vi "Get SubpanelVI Info.vi"(8 "error in (no error)":errorcluster, 11 "Motor Configuration in":refnum<class "LogicIO Configuration.lvclass">) -> (0 "error out":errorcluster, 1 "Subpanel VI data":T1, 2 "Category string":string, 3 "Motor Configuration out":refnum<class "LogicIO Configuration.lvclass">)   [LabVIEW 2016, in "Hardware.lvlib" / "LogicIO.lvlib" / "LogicIO Configuration.lvclass"]
uses:
  <userlib>/Common Components/Hardware/LogicIO/LogicIO Config/LogicIO Configuration.lvclass
  <userlib>/Configuration Dialog Actor/Methods/Data Retrieved by Lookup Table.ctl
  <userlib>/Configuration Dialog Actor/Configuration.lvclass
  <userlib>/Common Components/Hardware/LogicIO/LogicIO Config/LogicIO Configuration.lvclass/LogicIO Configuration.ctl
  <userlib>/Common Components/Hardware/Abstract Hardware/Hardware.lvclass/Hardware.ctl
  <userlib>/Common Components/Hardware/Abstract Hardware/Read Label.vi
  <userlib>/Common Components/Hardware/LogicIO/LogicIO/LogicIO.lvclass
  C:/Program Files (x86)/National Instruments/LabVIEW 2016/user.lib/Common Components/Hardware/Abstract Hardware/Hardware.lvclass
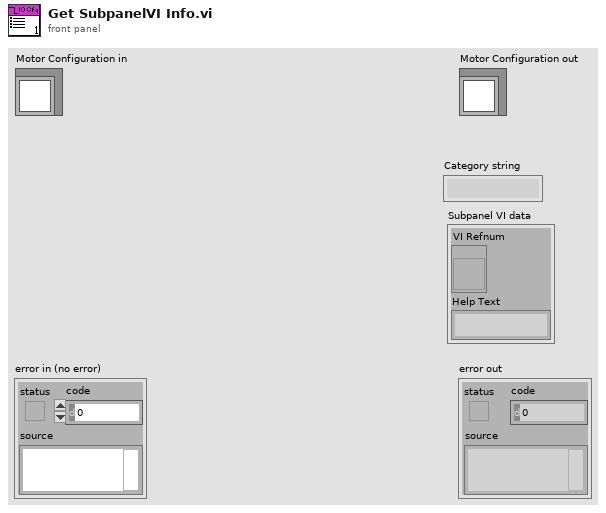
[diagram p1: front panel]
types:
  T1 = typedef "Configuration.lvlib/Configuration.lvclass/Data Retrieved by Lookup Table.ctl" = cluster{"VI Refnum":refnum<vi>, "Help Text":string}
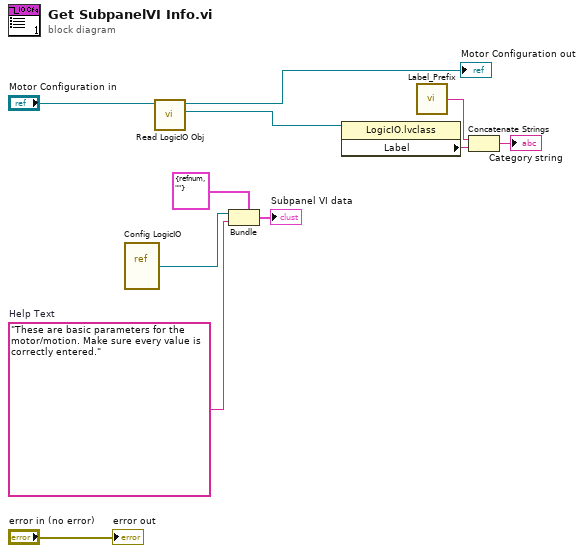
[diagram p0: block diagram]
diagram:
  w3 = "These are basic parameters for the motor/motion. Make sure every value is correctly entered."  # Help Text
  n1 = vi-ref <userlib>:"Config LogicIO.vi"() -> (w4:refnum<vi>)
  n2 = call <userlib>:"Read LogicIO Obj.vi"("LogicIO Configuration in"="Motor Configuration in") -> ("Hardware.lvlib:LogicIO.lvlib:LogicIO.lvclass"=w9:refnum<class "LogicIO.lvclass">, "LogicIO Configuration out"=→"Motor Configuration out":refnum<class "LogicIO Configuration.lvclass">)  [unwired: 9 in]
  n3 = Bundle(cluster=T1 {"VI Refnum"=refnum, "Help Text"=""} ("output cluster"), "VI Refnum"=w4, "Help Text"=w3) -> (→"Subpanel VI data":T1)
  n4 = property class="LogicIO.lvclass"(reference=w9) -> ("Label"=w1:string)  [unwired: 1 in, 2 out]
  n5 = call <userlib>:"Label_Prefix.vi"() -> ("Label Prefix String"=w10:string)
  n6 = Concatenate Strings(w10, w1) -> (→"Category string":string)
  "error out" <- "error in (no error)"
